vi "Panel_Manipulation.vi"() -> ()   [LabVIEW 2014]
uses:
  <vilib>/Utility/miscctls.llb/LVRectTypeDef.ctl
  <vilib>/Utility/miscctls.llb/LVPositionTypeDef.ctl
panel:
  in  "Position":T1
  out "Tab Control":enum32{"Setup", "Waiting", "Access", "Denied"}(tab)
  in  "Front Panel Window:Panel Bounds":T2={"Left"=0, "Top"=0, "Right"=500, "Bottom"=500}
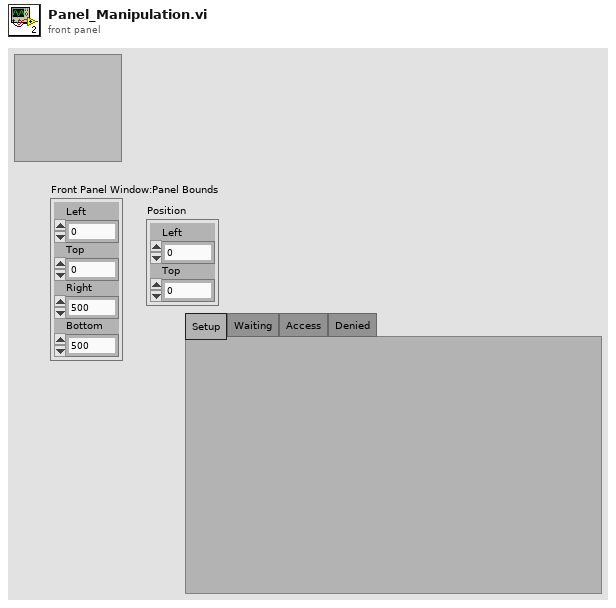
[diagram p1: front panel]
types:
  T1 = typedef "LVPositionTypeDef.ctl" = cluster{"Left":i32, "Top":i32}
  T2 = typedef "LVRectTypeDef.ctl" = cluster{"Left":i16, "Top":i16, "Right":i16, "Bottom":i16}
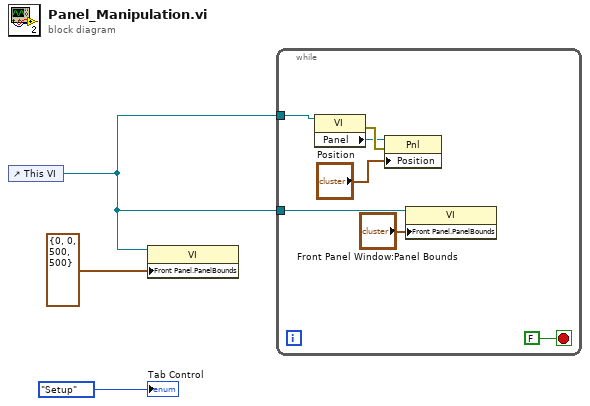
[diagram p0: block diagram]
diagram:
  n1 = control-ref of="This VI"() -> (w1:refnum<vi>)
  n2 = property class="VI"(reference=w1, "Front Panel.PanelBounds"=T2 {"Left"=0, "Top"=0, "Right"=500, "Bottom"=500} ("Front Panel Window:Panel Bounds 2")) -> ()  [unwired: 1 in, 2 out]
  n3 = while {
    tunnel: w1 -> [w9]
    tunnel: w1 -> [w5]
    stop <- FALSE stop-if-true
    n4 = property class="VI"(reference=w5) -> (error out=w7:errorcluster, "Panel"=w6:refnum<vi>)  [unwired: 1 in, 1 out]
    n5 = property class="Pnl"(reference=w6, error in=w7, "Position"="Position") -> ()  [unwired: 2 out]
    n6 = property class="VI"(reference=w9, "Front Panel.PanelBounds"="Front Panel Window:Panel Bounds") -> ()  [unwired: 1 in, 2 out]
  }
  "Tab Control" <- enum32{"Setup", "Waiting", "Access", "Denied"}."Setup" ("Tab Control 2")
